vi "Virtual Spring.vi"(9 "P Gain":dbl[](array[numeric])=[50.0, 50.0], 10 "Reference Position":dbl[](array[numeric]), 11 "Actual Position":dbl[](array[numeric])) -> (3 "Desired Force Matrix":T1)   [LabVIEW 2021]
uses:
  <vilib>/Analysis/Matrix/Datatypes/RealMatrix.ctl
  <vilib>/Analysis/Matrix/Numeric/Conversions/Array To Matrix - RA.vi
  <vilib>/Analysis/Matrix/NI_Matrix.lvlib
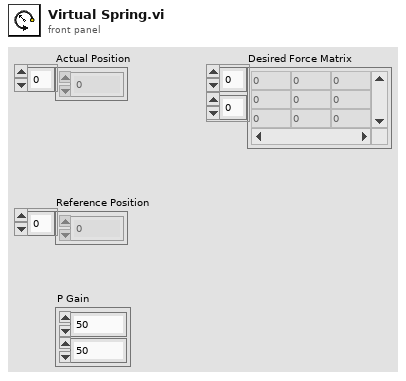
[diagram p1: front panel]
types:
  T1 = typedef "NI_Matrix.lvlib/RealMatrix.ctl" = dbl[][]
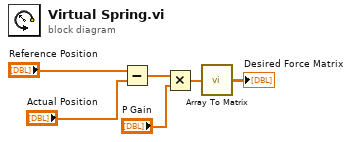
[diagram p0: block diagram]
diagram:
  n1 = Subtract(x="Reference Position", y="Actual Position") -> (x-y=w1:dbl[])
  n2 = Multiply(x=w1, y="P Gain") -> (x*y=w2:dbl[])
  n3 = call-poly <vilib>:"Array To Matrix.vi"("Real 1D Array"=w2) -> ("Real Matrix (Column Vector)"=→"Desired Force Matrix":T1)
